vi "PortInit2nd.vi"(1 "PortNumber":i32=11) -> (0 "Done":bool)   [LabVIEW 2013]
panel:
  in  "Baud rate XY":u32=38400
  # "Port Number 0=COM1"
  # "Initialize Serial Port.\nDefault setting is 38400/8N1/None."
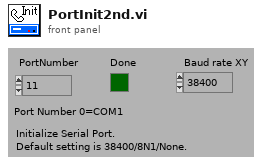
[diagram p1: front panel]
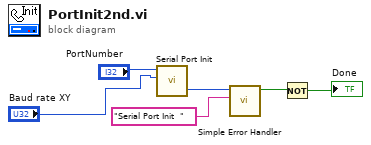
[diagram p0: block diagram]
diagram:
  n1 = call <vilib>:"Serial Port Init.vi"("baud rate"="Baud rate XY", "port number"="PortNumber") -> ("error code"=w5:i32)  [unwired: 5 in]
  n2 = call <vilib>:"Simple Error Handler.vi"("error code (no error:0)"=w5, "error source (\" \")"="Serial Port Init  ") -> ("error?"=w4:bool)  [unwired: 2 in, 5 out]
  n3 = Not(x=w4) -> (.not. x?=→"Done":bool)
